vi "Error Query.vi"(7 "bridge error to error out? (F)":bool, 8 "error in (no error)":errorcluster, 9 "firmware revision":string(combo), 10 "measurement line":string, 11 "VISA resource name":refnum<visa-resource-name>) -> (0 "error out":errorcluster, 2 "bridge error":T1, 3 "VISA resource name out":refnum<visa-resource-name>)   [LabVIEW 2025, in "Andeen-Hagerling 2700A.lvlib"]
doc: "Checks bridge results for an error code. If there isan error it will be included in the error out signal depending on the state of the bridge error to error out parameter. It may not be desirable to include a bridge error in the error out signal because that will preclude any further Visa operations until there error is cleared, and many bridge errors represent soft error conditions."
uses:
  Andeen-Hagerling 2700A.lvlib
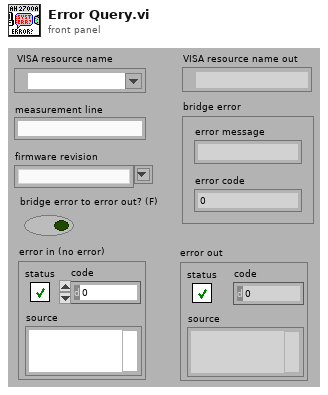
[diagram p1: front panel]
types:
  T1 = cluster{"error message":string, "error code":i32}
  T2 = cluster{"error code":i32, "frequency":dbl, "capacitance":dbl, "loss":dbl, "greater than":bool, "voltage":dbl}
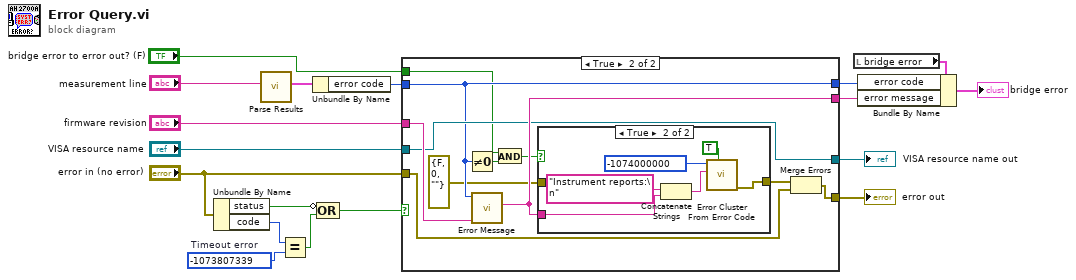
[diagram p0: block diagram]
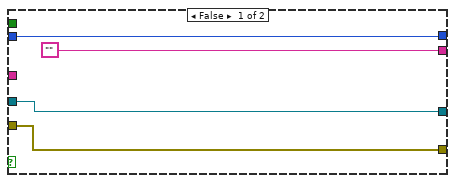
[diagram p2: hidden frame]
diagram:
  w13 = -1073807339  # Timeout error
  n1 = Unbundle By Name("error in (no error)") -> ("status"=w14:bool, "code"=w11:i32)
  n2 = call "Parse Results.vi"("measurement line"="measurement line") -> ("measurement results"=w6:T2)  [unwired: 9 in]
  n3 = Equal?(x=w11, y=w13) -> (x = y?=w12:bool)
  n4 = Unbundle By Name(w6) -> ("error code"=w7:i32)
  n5 = Compound Arithmetic op=OR(invert w14, w12) -> (w10:bool)
  n6 = case shown="True" w10 {
    tunnel: [w22 w28] -> w18
    tunnel: "VISA resource name" -> [w22 w28]
    tunnel: "error in (no error)" -> [w21 w31]
    tunnel: [w21 w33] -> w16
    tunnel: ["" w30] -> w3
    tunnel: [w19 w27] -> w4
    tunnel: "firmware revision" -> [_ w29]
    tunnel: w7 -> [w19 w27]
    tunnel: "bridge error to error out? (F)" -> [_ w23]
    frame False {
    }
    frame True {
      n7 = Not Equal To 0?(x=w27) -> (x != 0?=w24:bool)
      n8 = call "Error Message.vi"("firmware revision"=w29, "error number"=w27) -> ("error message"=w30:string)  [unwired: 9 in]
      n9 = And(x=w23, y=w24) -> (x .and. y?=w25:bool)
      n10 = case shown="True" w25 {
        tunnel: w30 -> [_ w39]
        tunnel: [w34 w35] -> w32
        tunnel: errorcluster {"status"=FALSE, "code"=0, "source"=""} ("error in (no error)") -> [w34 _]
        frame False {
        }
        frame True {
          n11 = Concatenate Strings("Instrument reports:\n" ("Source"), w39) -> (w36:string)
          n12 = call <vilib>:"Error Cluster From Error Code.vi"("show call chain? (False)"=TRUE, "error message (\"\")"=w36, "error code (0)"=-1074000000 ("Code")) -> ("error out"=w35:errorcluster)  [unwired: 6 in]
        }
      }
      n13 = Merge Errors(w32, w31) -> (w33:errorcluster)
    }
  }
  "VISA resource name out" <- w18
  "error out" <- w16
  n14 = local read "bridge error"() -> (w5:T1)
  n15 = Bundle By Name(cluster=w5, "error code"=w4, "error message"=w3) -> (→"bridge error":T1)
